vi "ConvertCoordinates.vi"(8 "error in (no error)":errorcluster, 9 "Spherical Coordinates In":cluster{"R":dbl, "Theta":dbl, "Phi":dbl}={"R"=nan, "Theta"=nan, "Phi"=nan}, 10 "Cylindrical Coordinates In":cluster{"Row":dbl, "Theta":dbl, "Z":dbl}={"Row"=nan, "Theta"=nan, "Z"=nan}, 11 "XYZ Coordinates In":cluster{"X":dbl, "Y":dbl, "Z":dbl}={"X"=nan, "Y"=nan, "Z"=nan}) -> (0 "error out":errorcluster, 1 "Spherical Coordinates Out":cluster{"R":dbl, "Theta":dbl, "Phi":dbl}={"R"=nan, "Theta"=nan, "Phi"=nan}, 2 "Cylindrical Coordinates Out":cluster{"Row":dbl, "Theta":dbl, "Z":dbl}={"Row"=nan, "Theta"=nan, "Z"=nan}, 3 "XYZ Coordinates Out":cluster{"X":dbl, "Y":dbl, "Z":dbl}={"X"=nan, "Y"=nan, "Z"=nan})   [LabVIEW 2019]
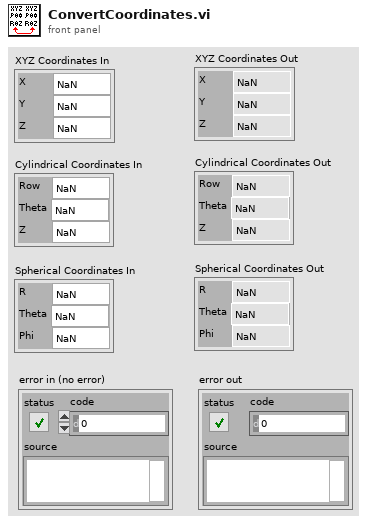
[diagram p1: front panel]
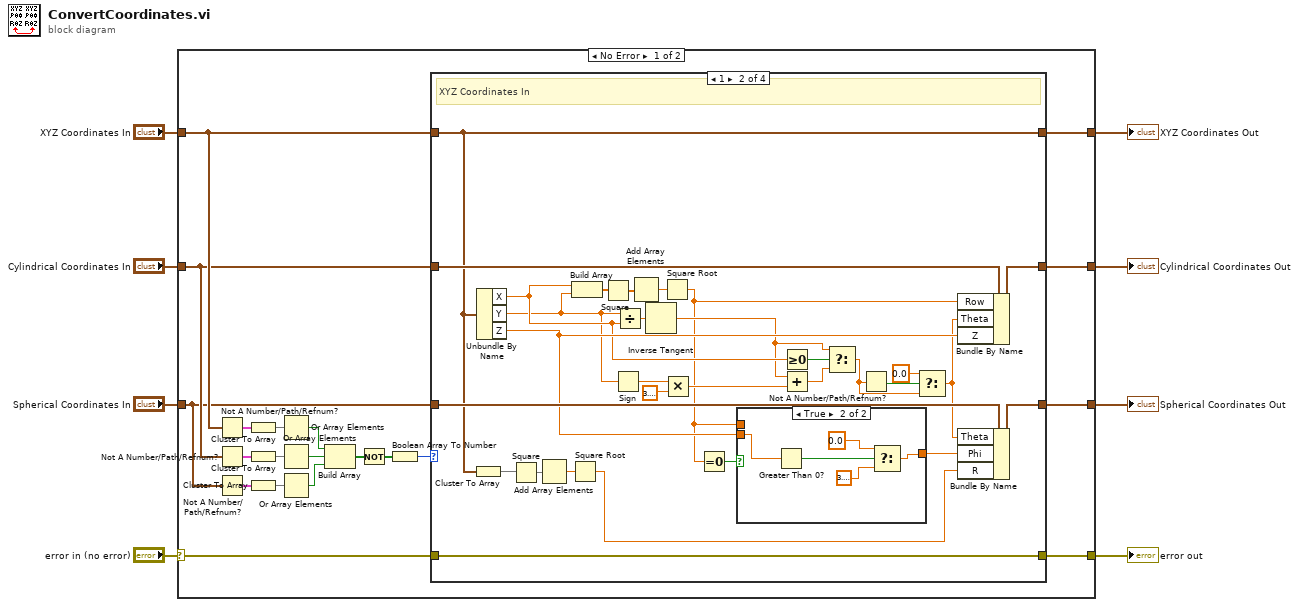
[diagram p0: block diagram]
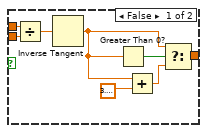
[diagram p3: hidden frame]
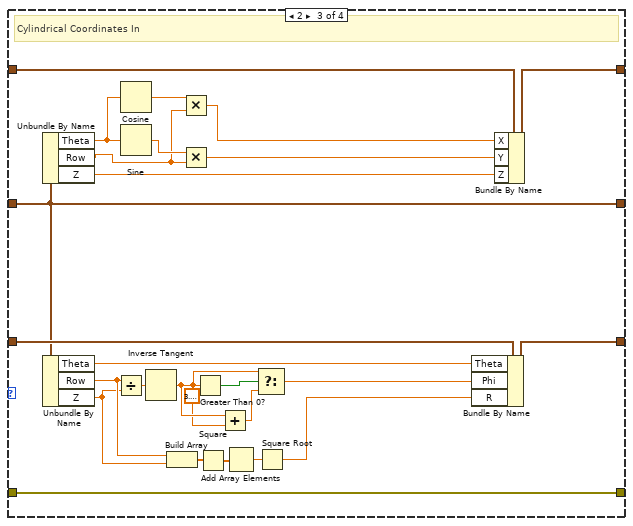
[diagram p4: hidden frame]
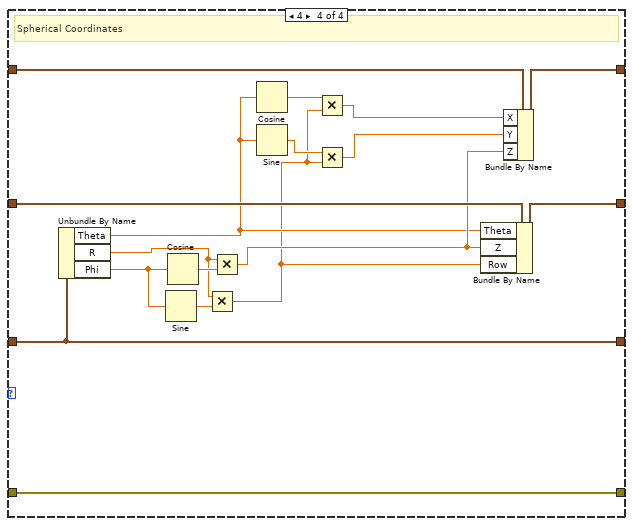
[diagram p5: hidden frame]
diagram:
  n1 = case shown="No Error" "error in (no error)" {
    selector: "error in (no error)" -> [w17 w122]
    tunnel: "XYZ Coordinates In" -> [w22 w120]
    tunnel: [w16 w122] -> w6
    tunnel: "Cylindrical Coordinates In" -> [w13 w121]
    tunnel: "Spherical Coordinates In" -> [w10 w119]
    tunnel: [w14 w120] -> w3
    tunnel: [w12 w121] -> w2
    tunnel: [w11 w119] -> w1
    frame No Error {
      n2 = Not A Number/Path/Refnum?(number/path/refnum=w22) -> (NaN/Path/Refnum?=w24:cluster{"X":bool, "Y":bool, "Z":bool})
      n3 = Not A Number/Path/Refnum?(number/path/refnum=w13) -> (NaN/Path/Refnum?=w25:cluster{"Row":bool, "Theta":bool, "Z":bool})
      n4 = Not A Number/Path/Refnum?(number/path/refnum=w10) -> (NaN/Path/Refnum?=w28:cluster{"R":bool, "Theta":bool, "Phi":bool})
      n5 = Cluster To Array(cluster=w24) -> (array=w23:bool[])
      n6 = Cluster To Array(cluster=w25) -> (array=w26:bool[])
      n7 = Cluster To Array(cluster=w28) -> (array=w27:bool[])
      n8 = Or Array Elements(Boolean array=w23) -> (logical OR=w21:bool)
      n9 = Or Array Elements(Boolean array=w26) -> (logical OR=w20:bool)
      n10 = Or Array Elements(Boolean array=w27) -> (logical OR=w19:bool)
      n11 = Build Array(w21, w20, w19) -> (w18:bool[])
      n12 = Not(x=w18) -> (.not. x?=w9:bool[])
      n13 = Boolean Array To Number(Boolean array=w9) -> (number=w15:u32)
      n14 = case shown="1" w15 {
        tunnel: w22 -> [w31 w51 w85 w116]
        tunnel: w17 -> [w32 w59 w96 w118]
        tunnel: [w32 w59 w96 w118] -> w16
        tunnel: [w31 w51 w93 w115] -> w14
        tunnel: [w30 w57 w84 w114] -> w12
        tunnel: w13 -> [w30 w58 w84 w117]
        tunnel: [w29 w55 w94 w113] -> w11
        tunnel: w10 -> [w29 w56 w95 w113]
        frame Default {
          # "ERROR"
        }
        frame 1 {
          # "XYZ Coordinates In"
          n15 = Cluster To Array(cluster=w51) -> (array=w48:dbl[])
          n16 = Unbundle By Name(w51) -> ("X"=w44:dbl, "Y"=w42:dbl, "Z"=w54:dbl)
          n17 = Square(x=w48) -> (x^2=w49:dbl[])
          n18 = Add Array Elements(numeric array=w49) -> (sum=w50:dbl)
          n19 = Square Root(x=w50) -> (sqrt(x)=w47:dbl)
          n20 = Build Array(w44, w42) -> (w62:dbl[])
          n21 = Square(x=w62) -> (x^2=w61:dbl[])
          n22 = Sign(1:w42) -> (0:w40:dbl)
          n23 = Divide(x=w42, y=w44) -> (x/y=w52:dbl)
          n24 = Add Array Elements(numeric array=w61) -> (sum=w60:dbl)
          n25 = Inverse Tangent(1:w52) -> (0:w43:dbl)
          n26 = Square Root(x=w60) -> (sqrt(x)=w34:dbl)
          n27 = Multiply(x=w40, y=3.141592653589793) -> (x*y=w39:dbl)
          n28 = Equal To 0?(x=w34) -> (x = 0?=w33:bool)
          n29 = case shown="True" w33 {
            tunnel: w54 -> [w66 w75]
            tunnel: [w65 w74] -> w53
            tunnel: w34 -> [w63 _]
            frame False {
              n30 = Divide(x=w63, y=w66) -> (x/y=w67:dbl)
              n31 = Inverse Tangent(1:w67) -> (0:w64:dbl)
              n32 = Greater Than 0?(x=w64) -> (x > 0?=w69:bool)
              n33 = Add(x=w64, y=3.141592653589793) -> (x+y=w70:dbl)
              n34 = Select(t=w64, s=w69, f=w70) -> (s? t:f=w65:dbl)
            }
            frame True {
              n35 = Greater Than 0?(x=w75) -> (x > 0?=w73:bool)
              n36 = Select(t=0.0, s=w73, f=3.141592653589793) -> (s? t:f=w74:dbl)
            }
          }
          n37 = Greater Or Equal To 0?(x=w44) -> (x >= 0?=w45:bool)
          n38 = Add(x=w43, y=w39) -> (x+y=w46:dbl)
          n39 = Select(t=w43, s=w45, f=w46) -> (s? t:f=w37:dbl)
          n40 = Not A Number/Path/Refnum?(number/path/refnum=w37) -> (NaN/Path/Refnum?=w38:bool)
          n41 = Select(t=0.0, s=w38, f=w37) -> (s? t:f=w35:dbl)
          n42 = Bundle By Name(cluster=w58, "Row"=w34, "Theta"=w35, "Z"=w54) -> (w57:cluster{"Row":dbl, "Theta":dbl, "Z":dbl})
          n43 = Bundle By Name(cluster=w56, "Theta"=w35, "Phi"=w53, "R"=w47) -> (w55:cluster{"R":dbl, "Theta":dbl, "Phi":dbl})
        }
        frame 2 {
          # "Cylindrical Coordinates In"
          n44 = Unbundle By Name(w84) -> ("Theta"=w81:dbl, "Row"=w78:dbl, "Z"=w82:dbl)
          n45 = Unbundle By Name(w84) -> ("Theta"=w91:dbl, "Row"=w87:dbl, "Z"=w83:dbl)
          n46 = Divide(x=w87, y=w83) -> (x/y=w97:dbl)
          n47 = Cosine(x=w81) -> (cos(x)=w79:dbl)
          n48 = Sine(x=w81) -> (sin(x)=w80:dbl)
          n49 = Inverse Tangent(1:w97) -> (0:w101:dbl)
          n50 = Build Array(w87, w83) -> (w90:dbl[])
          n51 = Multiply(x=w79, y=w78) -> (x*y=w77:dbl)
          n52 = Multiply(x=w80, y=w78) -> (x*y=w76:dbl)
          n53 = Greater Than 0?(x=w101) -> (x > 0?=w99:bool)
          n54 = Square(x=w90) -> (x^2=w89:dbl[])
          n55 = Add(x=w101, y=3.141592653589793) -> (x+y=w100:dbl)
          n56 = Add Array Elements(numeric array=w89) -> (sum=w88:dbl)
          n57 = Select(t=w101, s=w99, f=w100) -> (s? t:f=w92:dbl)
          n58 = Square Root(x=w88) -> (sqrt(x)=w86:dbl)
          n59 = Bundle By Name(cluster=w95, "Theta"=w91, "Phi"=w92, "R"=w86) -> (w94:cluster{"R":dbl, "Theta":dbl, "Phi":dbl})
          n60 = Bundle By Name(cluster=w85, "X"=w77, "Y"=w76, "Z"=w82) -> (w93:cluster{"X":dbl, "Y":dbl, "Z":dbl})
        }
        frame 4 {
          # "Spherical Coordinates"
          n61 = Unbundle By Name(w113) -> ("Theta"=w105:dbl, "R"=w109:dbl, "Phi"=w111:dbl)
          n62 = Sine(x=w111) -> (sin(x)=w110:dbl)
          n63 = Cosine(x=w111) -> (cos(x)=w112:dbl)
          n64 = Multiply(x=w109, y=w110) -> (x*y=w104:dbl)
          n65 = Multiply(x=w109, y=w112) -> (x*y=w108:dbl)
          n66 = Cosine(x=w105) -> (cos(x)=w106:dbl)
          n67 = Sine(x=w105) -> (sin(x)=w107:dbl)
          n68 = Multiply(x=w106, y=w104) -> (x*y=w103:dbl)
          n69 = Multiply(x=w107, y=w104) -> (x*y=w102:dbl)
          n70 = Bundle By Name(cluster=w117, "Theta"=w105, "Z"=w108, "Row"=w104) -> (w114:cluster{"Row":dbl, "Theta":dbl, "Z":dbl})
          n71 = Bundle By Name(cluster=w116, "X"=w103, "Y"=w102, "Z"=w108) -> (w115:cluster{"X":dbl, "Y":dbl, "Z":dbl})
        }
      }
    }
    frame Error {
    }
  }
  "XYZ Coordinates Out" <- w3
  "Cylindrical Coordinates Out" <- w2
  "Spherical Coordinates Out" <- w1
  "error out" <- w6
